vi "BLMove.vi"(0 "reference in":refnum<class "Redis.lvclass">, 5 "Source":string, 7 "Destination":string, 9 "WhereFrom":T1, 11 "Error In":errorcluster, 12 "WhereTo":T1, 13 "Timeout(1000ms)":i32=1000) -> (4 "reference out":refnum<class "Redis.lvclass">, 8 "Return":string, 15 "Error Out":errorcluster)   [LabVIEW 2020, in "Redis.lvclass"]
doc: "<b>LMOVE</b>\n\nBLMOVE is the blocking variant of LMOVE. When source contains elements, this command behaves exactly like LMOVE. When used inside a MULTI/EXEC block, this command behaves exactly like LMOVE. When source is empty, Redis will block the connection until another client pushes to it or until timeout (a double value specifying the maximum number of seconds to block) is reached. A timeout of zero can be used to block indefinitely.\n\nThis command comes in place of the now deprecated BRPOPLPUSH. Doing BLMOVE RIGHT LEFT is equivalent."
uses:
  Redis.lvclass
  Redis.lvclass/Redis.ctl
  SideEnum.ctl
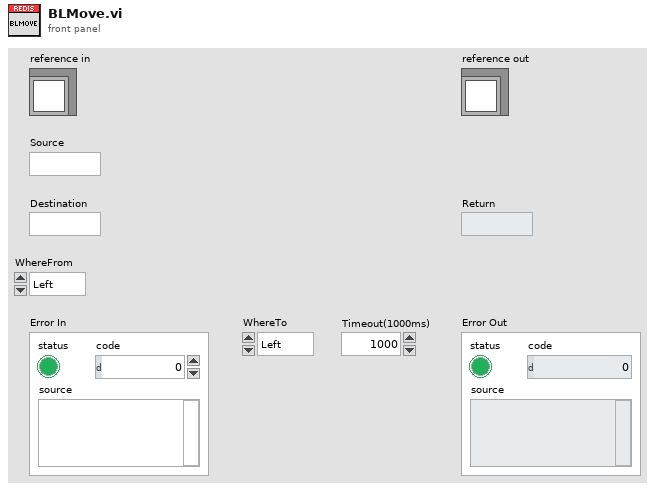
[diagram p1: front panel]
types:
  T1 = typedef "Redis.lvclass/SideEnum.ctl" = enum16{"Left", "Right"}
  T2 = typedef "Redis.lvclass/RedisDataType.ctl" = cluster{"Reply Type":T3, "Integer":i64, "String":string, "Multibulk":variant[], "StringData":string[]}
  T3 = typedef "Redis.lvclass/ReplyDataTypeEnum.ctl" = enum16{"None", "Error", "Status", "Nil", "Integer", "String", "Multibulk"}
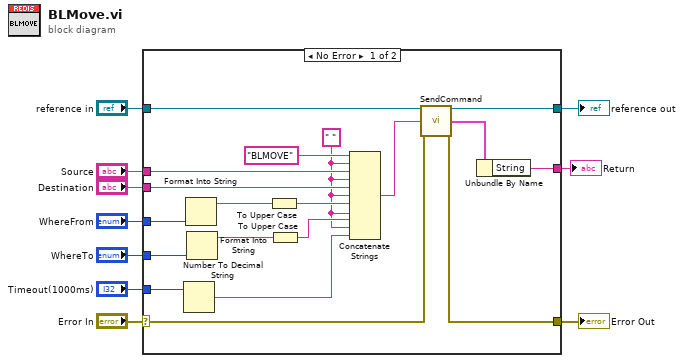
[diagram p0: block diagram]
diagram:
  n1 = case shown="No Error" "Error In" {
    selector: "Error In" -> [w27 w31]
    tunnel: [w26 w31] -> w9
    tunnel: [w29 w30] -> w7
    tunnel: "reference in" -> [w28 w30]
    tunnel: [w19 _] -> w4
    tunnel: "Source" -> [w23 _]
    tunnel: "WhereFrom" -> [w21 _]
    tunnel: "Destination" -> [w18 _]
    tunnel: "WhereTo" -> [w15 _]
    tunnel: "Timeout(1000ms)" -> [w13 _]
    frame No Error {
      w12 = " "
      n2 = Number To Decimal String(number=w13) -> (decimal integer string=w11:string)  [unwired: 1 in]
      n3 = Format Into String(w21) -> (resulting string=w20:string)  [unwired: 3 in, 1 out]
      n4 = Format Into String(w15) -> (resulting string=w16:string)  [unwired: 3 in, 1 out]
      n5 = To Upper Case(1:w20) -> (0:w17:string)
      n6 = To Upper Case(1:w16) -> (0:w14:string)
      n7 = Concatenate Strings("BLMOVE", w12, w23, w12, w18, w12, w17, w12, w14, w12, w11) -> (w22:string)
      n8 = call "SendCommand.vi"("reference in"=w28, "Command"=w22, "Error In"=w27) -> ("reference out"=w29:refnum<class "Redis.lvclass">, "Data"=w25:T2, "Error Out"=w26:errorcluster)  [unwired: 10 in]
      n9 = Unbundle By Name(w25) -> ("String"=w19:string)
    }
    frame Error {
    }
  }
  "Error Out" <- w9
  "reference out" <- w7
  "Return" <- w4
